vi "Register for Events.vi"(8 "error in (no error)":errorcluster, 11 "Samples in":refnum<class "Samples.lvclass">) -> (0 "error out":errorcluster, 2 "Event Registration Refnum":variant, 3 "Samples out":refnum<class "Samples.lvclass">)   [LabVIEW 2015, in "AMS UI.lvlib" / "Samples.lvclass"]
uses:
  Samples.lvclass
  eActor/eActor.lvclass/eActor.ctl
  Samples.lvclass/Samples.ctl
  eActor/eActor.lvclass
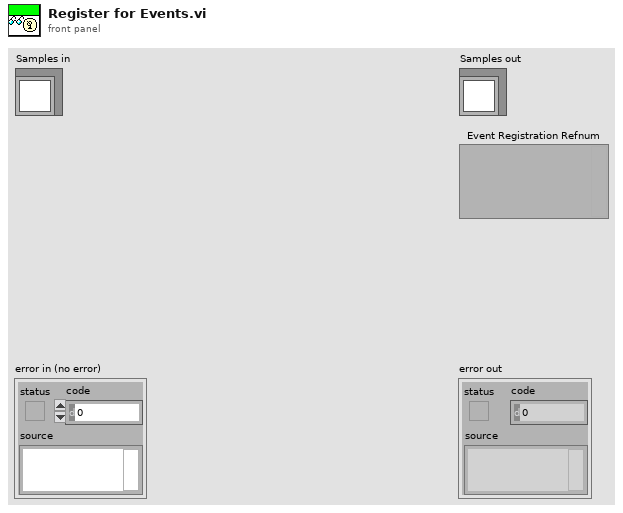
[diagram p1: front panel]
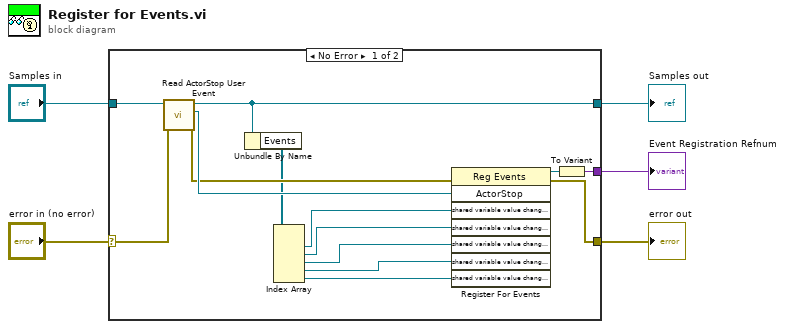
[diagram p0: block diagram]
diagram:
  n1 = case shown="No Error" "error in (no error)" {
    selector: "error in (no error)" -> [w15 w21]
    tunnel: [w12 w21] -> w4
    tunnel: "Samples in" -> [w19 w20]
    tunnel: [w18 w20] -> w2
    tunnel: [w16 _] -> w1
    frame No Error {
      n2 = call "Read ActorStop User Event.vi"("error in (no error)"=w15, "eActor in"=w19) -> ("error out"=w13:errorcluster, "ActorStop"=w14:refnum<user-event>, "eActor out"=w18:refnum<class "Samples.lvclass">)  [unwired: 7 in]
      n3 = Unbundle By Name(w18) -> ("Events"=w11:refnum<user-event>[])
      n4 = Index Array(array=w11) -> (element #1=w6:refnum<user-event>, element #2=w7:refnum<user-event>, element #3=w8:refnum<user-event>, element #4=w9:refnum<user-event>, element #5=w10:refnum<user-event>)  [unwired: 5 in]
      n5 = register-events(error in=w13, w14, w6, w7, w8, w9, w10) -> (reference out=w17:refnum<event-registration>, error out=w12:errorcluster)  [unwired: 1 in]
      n6 = To Variant(anything=w17) -> (Variant=w16:variant)
    }
    frame Error {
    }
  }
  "error out" <- w4
  "Samples out" <- w2
  "Event Registration Refnum" <- w1
